vi "instantiate_pdf_datasource.vi"(8 "error in (no error)":errorcluster, 10 "file_list":path[](array[path]), 11 "llm":refnum<class "abstract_llm_base.lvclass">) -> (0 "error out":errorcluster, 3 "datasource_pdf out":refnum<class "datasource_pdf.lvclass">)   [LabVIEW 2020, in "datasource_pdf.lvclass"]
uses:
  datasource_pdf.lvclass
  models/abstract_llm_base/abstract_llm_base.lvclass
  datasource_pdf.lvclass/datasource_pdf.ctl
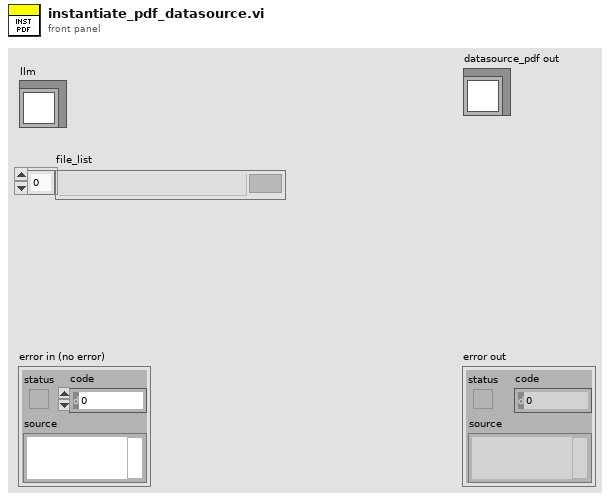
[diagram p1: front panel]
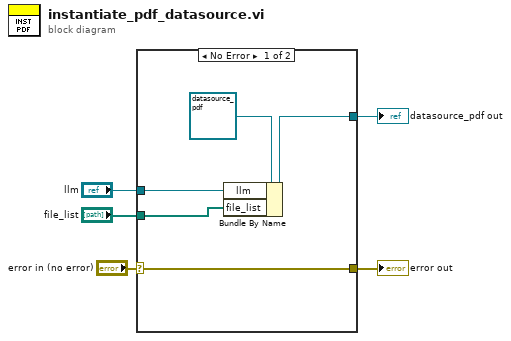
[diagram p0: block diagram]
diagram:
  n1 = case shown="No Error" "error in (no error)" {
    selector: "error in (no error)" -> [w10 w11]
    tunnel: [w10 w11] -> w4
    tunnel: [w6 _] -> w3
    tunnel: "llm" -> [w9 _]
    tunnel: "file_list" -> [w8 _]
    frame No Error {
      n2 = Bundle By Name(cluster=refnum<class "datasource_pdf.lvclass"> refnum ("datasource_pdf in"), "llm"=w9, "file_list"=w8) -> (w6:refnum<class "datasource_pdf.lvclass">)
    }
    frame Error {
    }
  }
  "error out" <- w4
  "datasource_pdf out" <- w3
